vi "Strip to Directory.vi"(8 "Error In":errorcluster, 11 "Path in":path) -> (0 "Error Out":errorcluster, 3 "Directory Out":path)   [LabVIEW 2016]
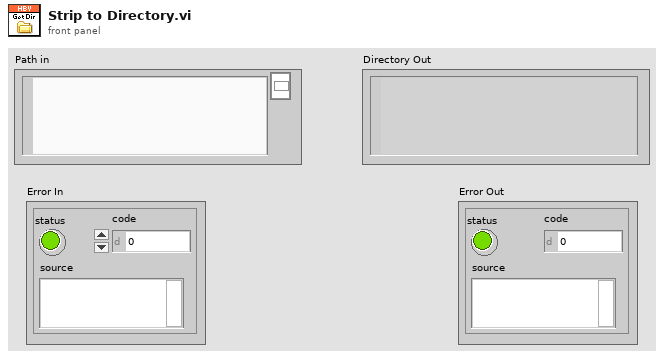
[diagram p1: front panel]
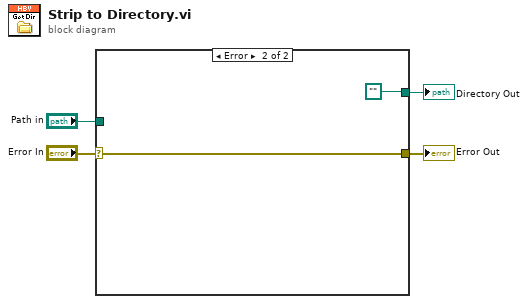
[diagram p0: block diagram]
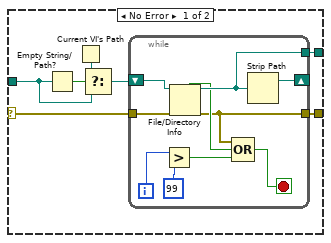
[diagram p2: hidden frame]
diagram:
  n1 = case shown="Error" "Error In" {
    selector: "Error In" -> [w5 w22]
    tunnel: [w11 w22] -> w4
    tunnel: [w10 path ""] -> w3
    tunnel: "Path in" -> [w7 _]
    frame No Error {
      n2 = Empty String/Path?(string/path=w7) -> (empty?=w9:bool)
      n3 = Current VI's Path() -> (path=w8:path)
      n4 = Select(t=w8, s=w9, f=w7) -> (s? t:f=w6:path)
      n5 = while {
        shift-right: [w19] -> _
        shift-left: w6 -> [w20]
        tunnel: [w12] -> w11
        tunnel: w5 -> [w21]
        tunnel: [w18] -> w10
        i -> [w17]
        stop <- w13 stop-if-true
        n6 = Greater?(x=w17, y=99) -> (0:w15:bool)
        n7 = File/Directory Info(path=w20, error in=w21) -> (path out=w18:path, directory=w14:bool, error out=w12:errorcluster)  [unwired: 4 out]
        n8 = Compound Arithmetic op=OR(w12, w14, w15) -> (w13:bool)
        n9 = Strip Path(path=w18) -> (stripped path=w19:path)  [unwired: 1 out]
      }
    }
    frame Error {
    }
  }
  "Error Out" <- w4
  "Directory Out" <- w3
